vi "knock it over.vi"(8 "Refnum in":refnum<k33>) -> (0 "Refnum out":refnum<k33>)   [LabVIEW 2014]
uses:
  TeleopCmd.ctl
  CmdFlag.ctl
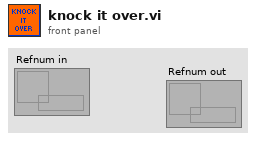
[diagram p1: front panel]
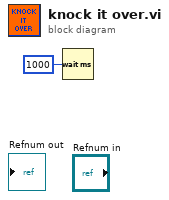
[diagram p0: block diagram]
diagram:
  n1 = Wait (ms)(milliseconds to wait=u32 1000) -> ()  [unwired: 1 out]
